vi "GetStaleStreamFilesFromDisk.vi"(6 "must contain block 0":bool, 8 "error in (no error)":errorcluster, 11 "data directory":path) -> (0 "error out":errorcluster, 1 "data group":string, 2 "stream id":string, 3 "file paths":path[](array[path]), 4 "files found":i32)   [LabVIEW 2017, in "FileManager.lvlib"]
uses:
  <vilib>/addons/InsightCM/Devices/Shared/Common/FileManager/FileManager.lvlib
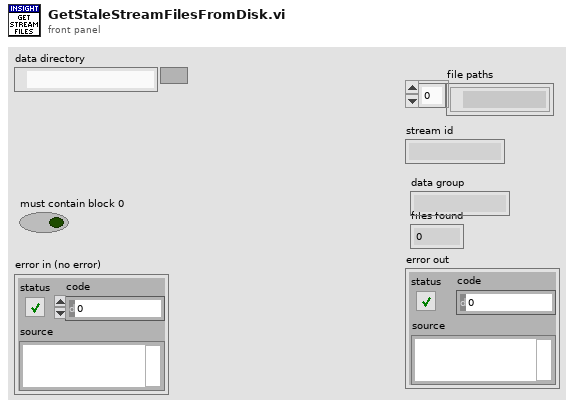
[diagram p1: front panel]
types:
  T1 = cluster{"last mod":timestamp, "appended path":path, string}
  T2 = cluster{"last mod":timestamp, "appended path":path, string}[]
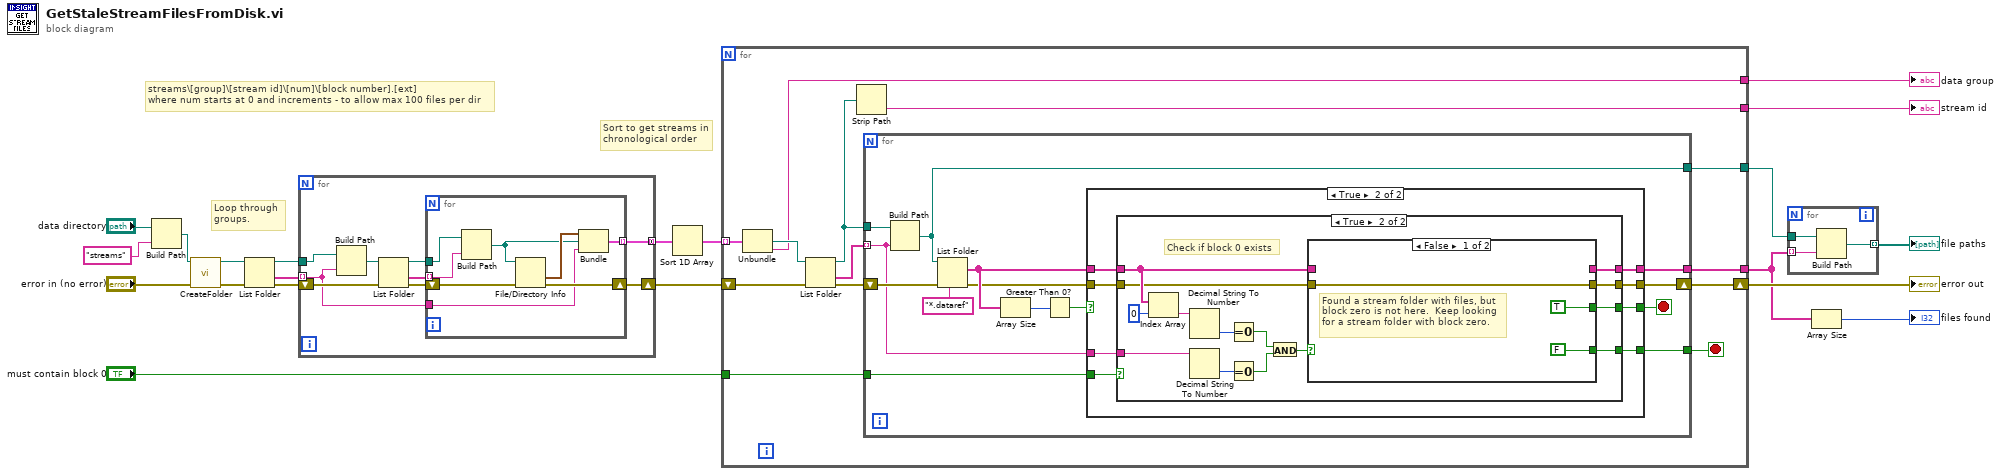
[diagram p0: block diagram]
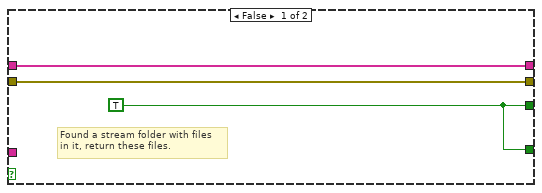
[diagram p3: hidden frame]
diagram:
  # "Sort to get streams in\nchronological order"
  # "Loop through\ngroups."
  # "streams\\[group]\\[stream id]\\[num]\\[block number].[ext]\nwhere num starts at 0 and increments - to allow max 100 files per dir"
  n1 = Build Path(base path="data directory", name or relative path="streams") -> (appended path=w18:path)
  n2 = call <vilib>:"CreateFolder.vi"("error in (no error)"="error in (no error)", "folder"=w18) -> ("error out"=w7:errorcluster, "folder out"=w6:path)  [unwired: 8 in]
  n3 = List Folder(path=w6, error in=w7) -> (path out=w3:path, folder names=w4:string[], error out=w5:errorcluster)  [unwired: 3 out]
  n4 = for {
    tunnel: [w29] -> w15 mode=concatenating
    shift-right: [w25] -> w13
    shift-left: w5 -> [w24]
    tunnel: w4 -> [w21] mode=indexing
    tunnel: w3 -> [w23]
    n5 = Build Path(base path=w23, name or relative path=w21) -> (appended path=w22:path)
    n6 = List Folder(path=w22, error in=w24) -> (path out=w27:path, folder names=w28:string[], error out=w26:errorcluster)  [unwired: 3 out]
    n7 = for {
      tunnel: w27 -> [w37]
      tunnel: w28 -> [w36] mode=indexing
      shift-right: [w32] -> w25
      shift-left: w26 -> [w35]
      tunnel: [w31] -> w29 mode=indexing
      tunnel: w21 -> [w30]
      n8 = Build Path(base path=w37, name or relative path=w36) -> (appended path=w33:path)
      n9 = File/Directory Info(path=w33, error in=w35) -> (last mod=w34:timestamp, error out=w32:errorcluster)  [unwired: 5 out]
      n10 = Bundle("last mod"=w34, "appended path"=w33, w30) -> (w31:T1)  [unwired: 1 in]
    }
  }
  n11 = Sort 1D Array(array=w15) -> (sorted array=w14:T2)
  n12 = for {
    tunnel: w14 -> [w49] mode=indexing
    shift-right: [w47] -> w10
    shift-left: w13 -> [w46]
    tunnel: [w44] -> w12
    tunnel: [w43] -> w8
    tunnel: "must contain block 0" -> [w42]
    tunnel: [w41] -> w2
    tunnel: [w39] -> w1
    stop <- w45 stop-if-true
    n13 = Unbundle(w49) -> ("appended path"=w48:path, w41:string)  [unwired: 1 out]
    n14 = List Folder(path=w48, error in=w46) -> (path out=w40:path, folder names=w38:string[], error out=w50:errorcluster)  [unwired: 3 out]
    n15 = Strip Path(path=w40) -> (name=w39:string)  [unwired: 1 out]
    n16 = for {
      tunnel: w38 -> [w52] mode=indexing
      tunnel: w40 -> [w64]
      tunnel: [w55] -> w44
      shift-right: [w54] -> w47
      shift-left: w50 -> [w63]
      tunnel: [w60] -> w43
      tunnel: [w53] -> w45
      tunnel: w42 -> [w61]
      stop <- w62 stop-if-true
      n17 = Build Path(base path=w64, name or relative path=w52) -> (appended path=w55:path)
      n18 = List Folder(path=w55, pattern="*.dataref", error in=w63) -> (filenames=w58:string[], error out=w57:errorcluster)  [unwired: 3 out]
      n19 = Array Size(array=w58) -> (size(s)=w51:i32)
      n20 = Greater Than 0?(x=w51) -> (x > 0?=w56:bool)
      n21 = case shown="True" w56 {
        selector: w56 -> [w65 _]
        tunnel: [w65 w75] -> w62
        tunnel: w61 -> [_ w74]
        tunnel: w58 -> [w67 w72]
        tunnel: [w67 w73] -> w60
        tunnel: [w66 w70] -> w54
        tunnel: w57 -> [w66 w71]
        tunnel: [w65 w69] -> w53
        tunnel: w52 -> [_ w68]
        frame False {
        }
        frame True {
          n22 = case shown="True" w74 {
            tunnel: [w76 w85] -> w75
            tunnel: w72 -> [w78 w89]
            tunnel: [w78 w88] -> w73
            tunnel: w71 -> [w77 w86]
            tunnel: [w77 w87] -> w70
            tunnel: [w76 w84] -> w69
            tunnel: w68 -> [_ w83]
            frame False {
              w76 = TRUE
              # "Found a stream folder with files\nin it, return these files."
            }
            frame True {
              # "Check if block 0 exists"
              n23 = Index Array(array=w89, index=0) -> (element=w91:string)
              n24 = Decimal String To Number(string=w91) -> (number=w90:i32)  [unwired: 2 in, 1 out]
              n25 = Decimal String To Number(string=w83) -> (number=w82:i32)  [unwired: 2 in, 1 out]
              n26 = Equal To 0?(x=w90) -> (x = 0?=w80:bool)
              n27 = Equal To 0?(x=w82) -> (x = 0?=w81:bool)
              n28 = And(x=w80, y=w81) -> (x .and. y?=w79:bool)
              n29 = case shown="False" w79 {
                selector: w79 -> [_ w96]
                tunnel: w89 -> [_ w98]
                tunnel: [_ w98] -> w88
                tunnel: [w95 w97] -> w87
                tunnel: w86 -> [w95 w97]
                tunnel: [TRUE w96] -> w85
                tunnel: [FALSE w96] -> w84
                frame False {
                  # "Found a stream folder with files, but\nblock zero is not here.  Keep looking\nfor a stream folder with block zero."
                }
                frame True {
                  # "Found a stream with block 0,\nsend these files."
                }
              }
            }
          }
        }
      }
    }
  }
  "error out" <- w10
  "stream id" <- w1
  "data group" <- w2
  n30 = for {
    tunnel: w12 -> [w101]
    tunnel: w8 -> [w100] mode=indexing
    tunnel: [w99] -> w11 mode=indexing
    n31 = Build Path(base path=w101, name or relative path=w100) -> (appended path=w99:path)
  }
  "file paths" <- w11
  n32 = Array Size(array=w8) -> (size(s)=→"files found":i32)
